vi "Configure Power.vi"(8 "error in (no error)":errorcluster, 10 "Power [dBm]":dbl, 11 "VNA-FieldFox in":refnum<class "VNA-FieldFox.lvclass">) -> (0 "error out":errorcluster, 3 "VNA-FieldFox out":refnum<class "VNA-FieldFox.lvclass">)   [LabVIEW 2020, in "VNA-FieldFox.lvclass"]
doc: "Configure the output power.\nThe power will be corrected to the nearest supported."
uses:
  VNA-FieldFox.lvclass
  C:/Sandbox/Git_Sandbox/WiSpry Test Framework source code (LV20)/WiSpry Test Framework/Instruments/Instrument.lvclass
  Instrument.lvclass/Instrument.ctl
  <instrlib>/Agilent N99XX Series/Agilent N99XX Series.lvlib
  Instrument.lvclass
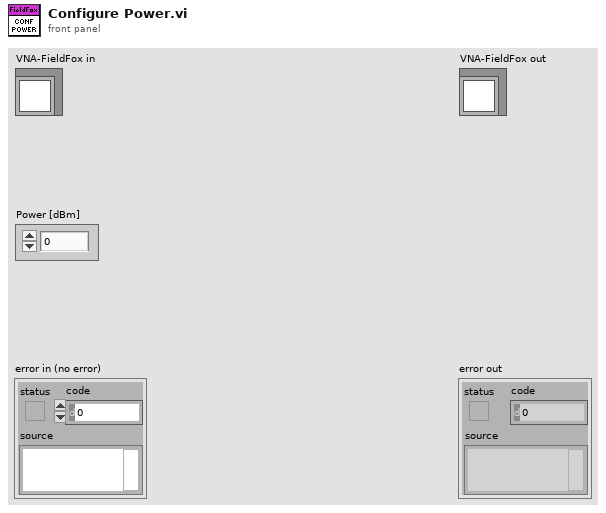
[diagram p1: front panel]
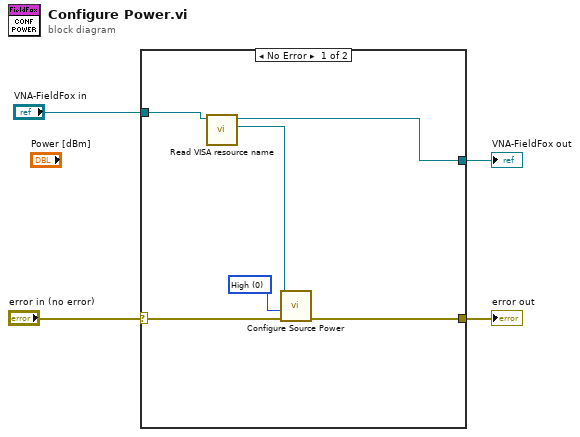
[diagram p0: block diagram]
diagram:
  n1 = case shown="No Error" "error in (no error)" {
    selector: "error in (no error)" -> [w10 w11]
    tunnel: [w9 w11] -> w3
    tunnel: "VNA-FieldFox in" -> [w8 w12]
    tunnel: [w6 w12] -> w1
    frame No Error {
      w5 = 0 items=["High", "Low", "Manually"] ("Power Type (0: High)")
      n2 = call "Read VISA resource name.vi"("Instrument in"=w8) -> ("VISA resource name"=w7:refnum<visa-resource-name>, "Instrument out"=w6:refnum<class "VNA-FieldFox.lvclass">)  [unwired: 9 in]
      n3 = call <instrlib>:"Configure Source Power.vi"("error in (no error)"=w10, "Power Type (0: High)"=w5, "VISA resource name"=w7) -> ("error out"=w9:errorcluster)  [unwired: 7 in, 1 out]
    }
    frame Error {
    }
  }
  "error out" <- w3
  "VNA-FieldFox out" <- w1
